vi "data_adjust.vi"(9 "数据高位":u8, 10 "数据低位":u8) -> (2 "瞬时加速度值":dbl)   [LabVIEW 2010]
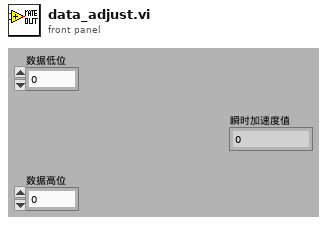
[diagram p1: front panel]
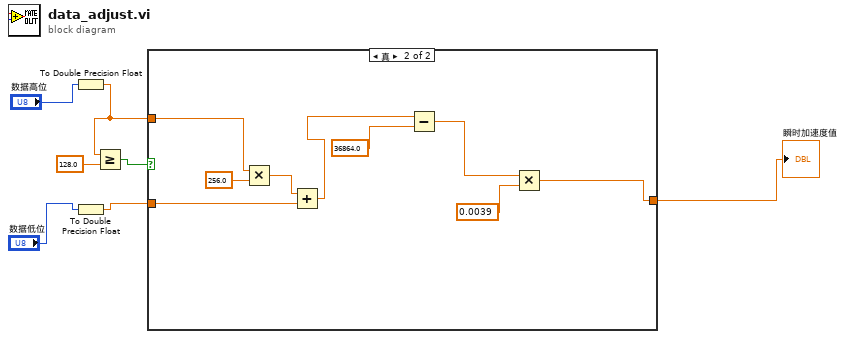
[diagram p0: block diagram]
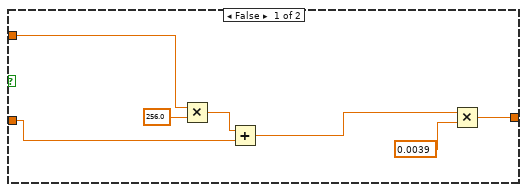
[diagram p2: hidden frame]
diagram:
  n1 = To Double Precision Float(number="数据高位") -> (double precision float=w4:dbl)
  n2 = To Double Precision Float(number="数据低位") -> (double precision float=w3:dbl)
  n3 = Greater Or Equal?(x=w4, y=128.0) -> (x >= y?=w7:bool)
  n4 = case shown="真" w7 {
    tunnel: w4 -> [w11 w23]
    tunnel: w3 -> [w10 w22]
    tunnel: [w8 w15] -> w1
    frame False {
      n5 = Multiply(x=w11, y=256.0) -> (x*y=w13:dbl)
      n6 = Add(x=w13, y=w10) -> (x+y=w9:dbl)
      n7 = Multiply(x=w9, y=0.0039) -> (x*y=w8:dbl)
    }
    frame True {
      n8 = Multiply(x=w23, y=256.0) -> (x*y=w20:dbl)
      n9 = Add(x=w20, y=w22) -> (x+y=w19:dbl)
      n10 = Subtract(x=w19, y=36864.0) -> (x-y=w17:dbl)
      n11 = Multiply(x=w17, y=0.0039) -> (x*y=w15:dbl)
    }
  }
  "瞬时加速度值" <- w1
